vi "GFG_core.vi"(0 "Variable Name in":string, 2 "Variant in":variant, 4 "Source VI":string, 5 "error in (no error)":errorcluster, 7 "Action":enum16{"Init", "Set", "Get", "Clear"}(ring)=enum."Get") -> (13 "Found/Replaced":bool, 14 "Variable Name Out":string, 15 "Data Type Out":T1, 16 "Variant Out":variant, 17 "All Variable Names Out":string[](array[string]), 18 "user event out":refnum<user-event>, 19 "error out":errorcluster)   [LabVIEW 2012]
doc: "This VI represents a functional global variable a.k.a. LV2 Global, which stores any data type as a variant. It was inspired by and adapted from a VI posted on the LabView Idea Exchange (http://forums.ni.com/t5/LabVIEW-Idea-Exchange/Generalized-Functional-Global-GFG/idi-p/1397744)"
uses:
  <vilib>/Utility/VariantDataType/Type.ctl
  <vilib>/Utility/VariantDataType/VariantType.lvlib
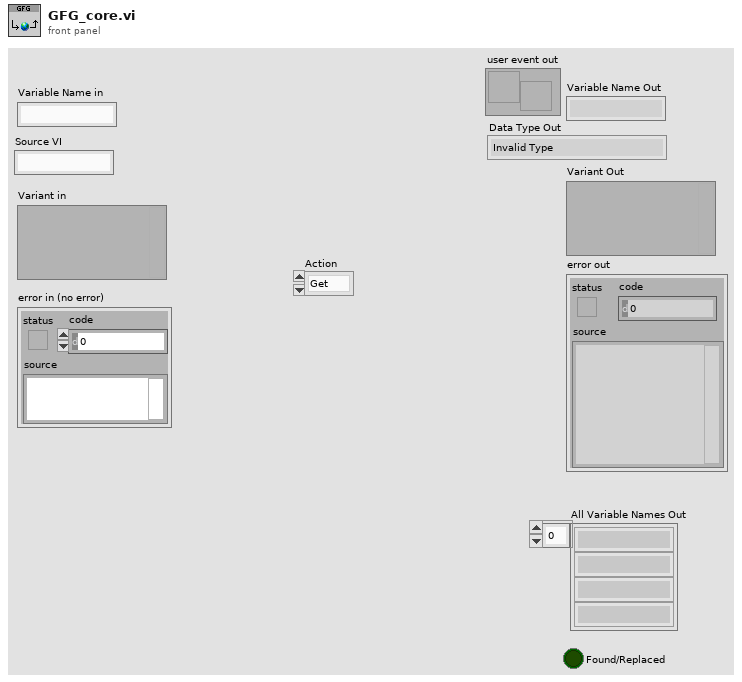
[diagram p1: front panel]
types:
  T1 = typedef "VariantType.lvlib/Type.ctl" = enum8{"Invalid Type", "Void", "I8", "I16", "I32", "I64", "U8", "U16", "U32", "U64", "Single Float", "Double Float", "Extended Float", "Single Complex", "Double Complex", "Extended Complex", "Enum U8", "Enum U16", "Enum U32", "Enum U64", "Single Float With Unit", "Double Float With Unit", "Extended Float With Unit", "Single Complex with Unit", "Double Complex with Unit", "Extended Complex with Unit", "Boolean", "String", "Path", "Picture", "Tag", "Array", "Cluster", "Variant", "LV Variant", "Waveform", "Timestamp", "Digital Waveform", "Digital Data", "ExpressData", "Refnum", "External Data", "VI", "Poly VI", "LabVIEW Class Instance", "Fixed Point"}
  T2 = cluster{"Source VI":string, "Variable Name":string, "Data Type":T1, "Variant":variant}
  T3 = enum16{"open", "replace", "create", "open or create", "replace or create", "replace or create with confirmation"}
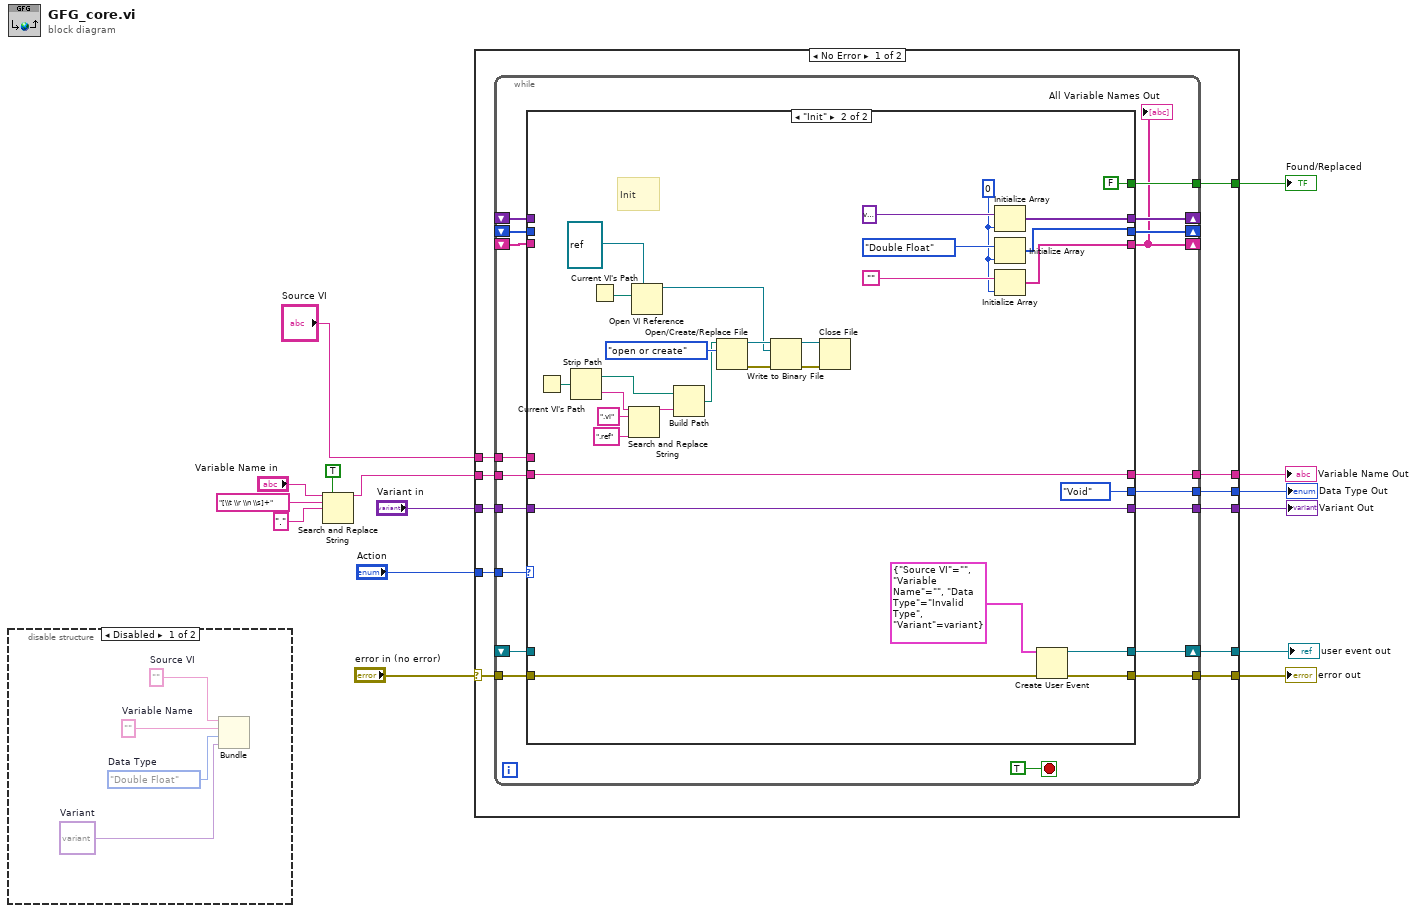
[diagram p0: block diagram]
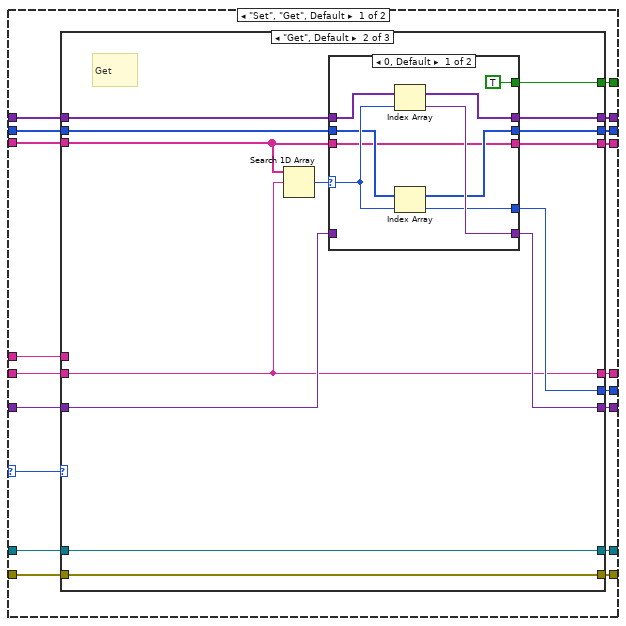
[diagram p3: hidden frame]
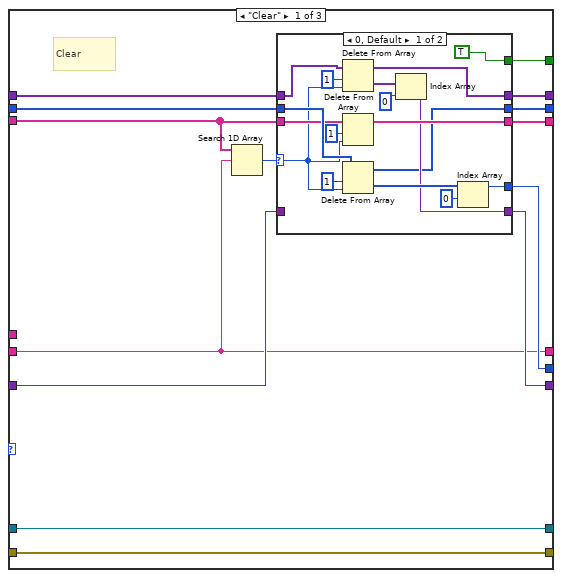
[diagram p4: hidden frame]
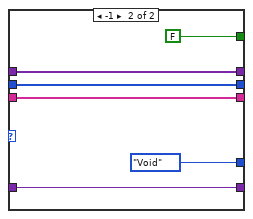
[diagram p5: hidden frame]
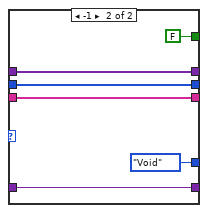
[diagram p6: hidden frame]
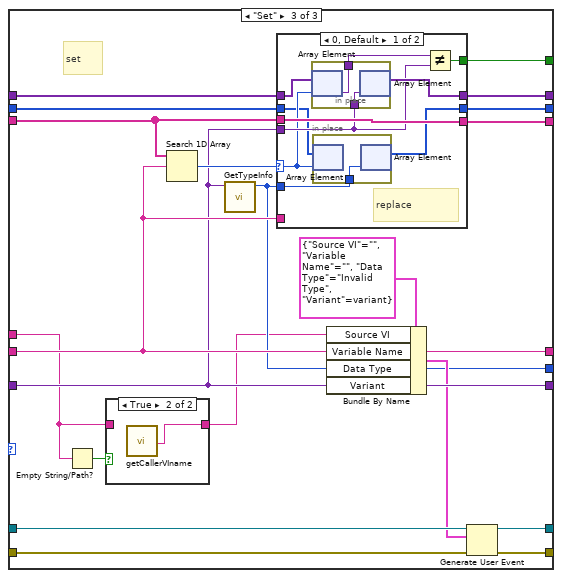
[diagram p7: hidden frame]
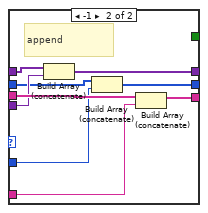
[diagram p9: hidden frame]
diagram:
  n1 = disable-structure shown="Disabled" {
    frame Disabled {
      w16 = variant(bool TRUE)  # Variant
      w18 = ""  # Variable Name
      w19 = ""  # Source VI
      w17 = Type."Double Float"  # Data Type
      n2 = Bundle("Source VI"=w19, "Variable Name"=w18, "Data Type"=w17, "Variant"=w16) -> ()  [unwired: 1 in, 1 out]
    }
    frame Enabled {
    }
  }
  n3 = Search and Replace String(replace all?=TRUE ("replace all? (F)"), input string="Variable Name in", search string="[\\t \\r \\n \\s]+", replace string="." ("replace string (\"\")")) -> (result string=w1:string)  [unwired: 4 in, 3 out]
  n4 = case shown="No Error" "error in (no error)" {
    selector: "error in (no error)" -> [w20 w208]
    tunnel: [w30 w207] -> w15
    tunnel: "Variant in" -> [w29 w207]
    tunnel: [w28 w208] -> w14
    tunnel: w1 -> [w25 w206]
    tunnel: "Source VI" -> [w27 _]
    tunnel: [w26 _] -> w12
    tunnel: [w24 _] -> w8
    tunnel: [w23 _] -> w7
    tunnel: [w22 w206] -> w10
    tunnel: "Action" -> [w21 _]
    frame No Error {
      n5 = while {
        tunnel: [w49] -> w30
        tunnel: w29 -> [w48]
        tunnel: w20 -> [w47]
        tunnel: [w46] -> w28
        tunnel: w25 -> [w44]
        shift-right: [w43] -> w23
        shift-left: _ -> [w42]
        tunnel: w27 -> [w41]
        shift-right: [w33] -> _
        shift-left: _ -> [w40]
        shift-right: [w39] -> _
        shift-left: _ -> [w38]
        tunnel: [w37] -> w26
        shift-right: [w36] -> _
        shift-left: _ -> [w35]
        tunnel: [w34] -> w24
        tunnel: [w32] -> w22
        tunnel: w21 -> [w31]
        stop <- TRUE stop-if-true
        n6 = case shown="\"Init\"" w31 {
          selector: w31 -> [w50 _]
          tunnel: [w60 w201] -> w49
          tunnel: w48 -> [w61 w201]
          tunnel: w47 -> [w65 w205]
          tunnel: [w64 w204] -> w46
          tunnel: w44 -> [w62 w197]
          tunnel: [w66 w196] -> w43
          tunnel: w42 -> [w67 _]
          tunnel: w41 -> [w63 _]
          tunnel: w40 -> [w59 _]
          tunnel: [w58 w203] -> w33
          tunnel: [w56 w200] -> w39
          tunnel: w38 -> [w57 _]
          tunnel: [w55 FALSE] -> w37
          tunnel: [w53 w202] -> w36
          tunnel: w35 -> [w54 _]
          tunnel: [w52 Type."Void" ("Type Enum")] -> w34
          tunnel: [w51 w197] -> w32
          frame "Set", "Get", Default {
            n7 = case shown="\"Get\", Default" w50 {
              tunnel: w67 -> [w81 w118 w151]
              tunnel: [w81 w118 w137] -> w66
              tunnel: w65 -> [w80 w117 w150]
              tunnel: [w80 w117 w132] -> w64
              tunnel: w63 -> [_ _ w134]
              tunnel: w62 -> [w70 w107 w141]
              tunnel: w61 -> [w76 w113 w140]
              tunnel: [w75 w112 w140] -> w60
              tunnel: w59 -> [w69 w106 w148]
              tunnel: [w68 w105 w147] -> w58
              tunnel: w57 -> [w78 w115 w146]
              tunnel: [w77 w114 w145] -> w56
              tunnel: [w74 w111 w144] -> w55
              tunnel: w54 -> [w73 w110 w143]
              tunnel: [w72 w109 w142] -> w53
              tunnel: [w71 w108 w136] -> w52
              tunnel: [w70 w107 w141] -> w51
              frame "Clear" {
                # "Clear"
                n8 = Search 1D Array(1D array=w69, element=w70) -> (index of element=w79:i32)  [unwired: 1 in]
                n9 = case shown="0, Default" w79 {
                  selector: w79 -> [w92 _]
                  tunnel: w78 -> [w98 w104]
                  tunnel: [w83 w104] -> w77
                  tunnel: w76 -> [_ w103]
                  tunnel: [w84 w103] -> w75
                  tunnel: [TRUE FALSE] -> w74
                  tunnel: w73 -> [w96 w102]
                  tunnel: [w82 w102] -> w72
                  tunnel: [w87 Type."Void" ("Data Type")] -> w71
                  tunnel: [w91 w101] -> w68
                  tunnel: w69 -> [w95 w101]
                  frame 0, Default {
                    n10 = Delete From Array(array=w98, length=1, index=w92) -> (deleted portion=w86:variant[], array with subset deleted=w83:variant[])
                    n11 = Delete From Array(array=w95, length=1, index=w92) -> (array with subset deleted=w91:string[])  [unwired: 1 out]
                    n12 = Delete From Array(array=w96, length=1, index=w92) -> (deleted portion=w89:T1[], array with subset deleted=w82:T1[])
                    n13 = Index Array(array=w86, index=0) -> (element=w84:variant)
                    n14 = Index Array(array=w89, index=0) -> (element=w87:T1)
                  }
                  frame -1 {
                  }
                }
              }
              frame "Get", Default {
                # "Get"
                n15 = Search 1D Array(1D array=w106, element=w107) -> (index of element=w116:i32)  [unwired: 1 in]
                n16 = case shown="0, Default" w116 {
                  selector: w116 -> [w122 _]
                  tunnel: w115 -> [w125 w131]
                  tunnel: [w125 w131] -> w114
                  tunnel: w113 -> [_ w130]
                  tunnel: [w124 w130] -> w112
                  tunnel: [TRUE FALSE] -> w111
                  tunnel: w110 -> [w121 w129]
                  tunnel: [w121 w129] -> w109
                  tunnel: [w120 Type."Void" ("Data Type")] -> w108
                  tunnel: [w119 w128] -> w105
                  tunnel: w106 -> [w119 w128]
                  frame 0, Default {
                    n17 = Index Array(array=w125, index=w122) -> (element=w124:variant)
                    n18 = Index Array(array=w121, index=w122) -> (element=w120:T1)
                  }
                  frame -1 {
                  }
                }
              }
              frame "Set" {
                # "set"
                n19 = Empty String/Path?(string/path=w134) -> (empty?=w135:bool)
                n20 = case shown="True" w135 {
                  tunnel: [w152 w153] -> w133
                  tunnel: w134 -> [w152 _]
                  frame False {
                  }
                  frame True {
                    n21 = call "getCallerVIname.vi"() -> ("VI name"=w153:string)  [unwired: 19 in]
                  }
                }
                n22 = Search 1D Array(1D array=w148, element=w141) -> (index of element=w149:i32)  [unwired: 1 in]
                n23 = call <vilib>:"GetTypeInfo.vi"("Variant"=w140) -> ("Type Enum"=w136:T1)  [unwired: 6 in, 4 out]
                n24 = case shown="0, Default" w149 {
                  selector: w149 -> [w157 _]
                  tunnel: w148 -> [w163 w175]
                  tunnel: [w163 w174] -> w147
                  tunnel: w146 -> [w162 w172]
                  tunnel: w141 -> [_ w173]
                  tunnel: w140 -> [w159 w171]
                  tunnel: [w161 w170] -> w145
                  tunnel: [w158 _] -> w144
                  tunnel: w143 -> [w156 w169]
                  tunnel: w136 -> [w154 w167]
                  tunnel: [w155 w168] -> w142
                  frame 0, Default {
                    # "replace"
                    n25 = in-place {
                      in-place-border: [w166] -> w160
                      in-place-border: w159 -> [w165]
                      n26 = in-place-array #1(w162, w157) -> (w166:variant)
                      n27 = in-place-array #1(w165) -> (w161:variant[])  [unwired: 1 out]
                    }
                    n28 = in-place {
                      in-place-border: w154 -> [w164]
                      n29 = in-place-array #2(w156, w157) -> ()  [unwired: 1 out]
                      n30 = in-place-array #2(w164) -> (w155:T1[])  [unwired: 1 out]
                    }
                    n31 = Not Equal?(x=w160, y=w159) -> (x != y?=w158:bool)
                  }
                  frame -1 {
                    # "append"
                    n32 = Build Array (concatenate)(w172, w171) -> (w170:variant[])
                    n33 = Build Array (concatenate)(w169, w167) -> (w168:T1[])
                    n34 = Build Array (concatenate)(w175, w173) -> (w174:string[])
                  }
                }
                n35 = Bundle By Name(cluster=T2 {"Source VI"="", "Variable Name"="", "Data Type"=enum."Invalid Type", "Variant"=variant} ("output cluster"), "Source VI"=w133, "Variable Name"=w141, "Data Type"=w136, "Variant"=w140) -> (w138:T2)
                n36 = Generate User Event(user event=w151, event data cluster=w138, error in=w150) -> (user event out=w137:refnum<user-event>, error out=w132:errorcluster)
              }
            }
          }
          frame "Init" {
            w192 = 0 ("dimension size")
            # "Init"
            n37 = Current VI's Path() -> (path=w190:path)
            n38 = Strip Path(path=w190) -> (stripped path=w186:path, name=w189:string)
            n39 = Current VI's Path() -> (path=w178:path)
            n40 = Search and Replace String(input string=w189, search string=".vi", replace string=".ref" ("replace string (\"\")")) -> (result string=w185:string)  [unwired: 5 in, 3 out]
            n41 = Open VI Reference(type specifier VI Refnum (for type only)=refnum<vi> refnum ("application reference (local)"), vi path=w178) -> (vi reference=w176:refnum<vi>)  [unwired: 4 in, 1 out]
            n42 = Build Path(base path=w186, name or relative path=w185) -> (appended path=w179:path)
            n43 = Open/Create/Replace File(file path (use dialog)=w179, operation (0:open)=T3."open or create") -> (refnum out=w182:refnum<file>, error out=w181:errorcluster)  [unwired: 4 in, 1 out]
            n44 = Write to Binary File(file (use dialog)=w182, data=w176, error in=w181) -> (refnum out=w183:refnum<file>, error out=w184:errorcluster)  [unwired: 3 in, 1 out]
            n45 = Close File(refnum=w183, error in=w184) -> ()  [unwired: 2 out]
            n46 = Initialize Array(variant ("Variant"), w192) -> (w200:variant[])
            n47 = Initialize Array(Type."Double Float" ("Data Type"), w192) -> (w202:T1[])
            n48 = Initialize Array("" ("Empty String Constant"), w192) -> (w203:string[])
            n49 = Create User Event(user event datatype=T2 {"Source VI"="", "Variable Name"="", "Data Type"=enum."Invalid Type", "Variant"=variant} ("output cluster"), error in=w205) -> (user event=w196:refnum<user-event>, error out=w204:errorcluster)
          }
        }
        "All Variable Names Out" <- w33
      }
    }
    frame Error {
    }
  }
  "Variant Out" <- w15
  "error out" <- w14
  "Found/Replaced" <- w12
  "Variable Name Out" <- w10
  "Data Type Out" <- w8
  "user event out" <- w7
